vi "난수플롯이벤트.vi"() -> ()   [LabVIEW 2014]
panel:
  in  "정지":bool
  out "웨이브폼 차트":dbl(graph)
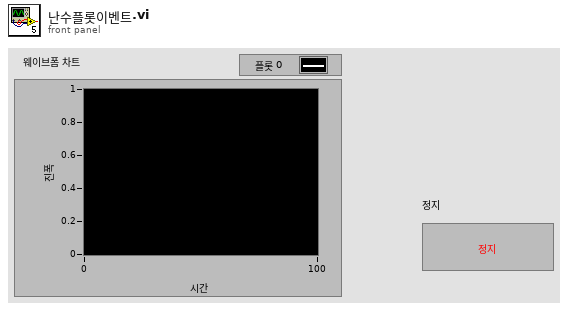
[diagram p1: front panel]
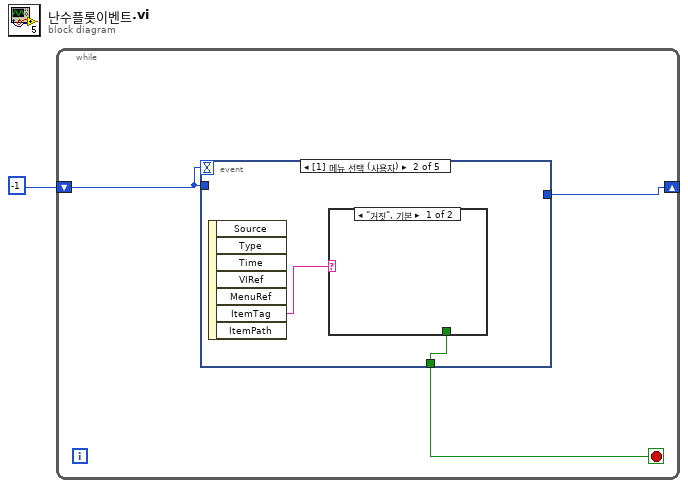
[diagram p0: block diagram]
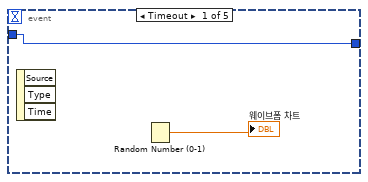
[diagram p2: hidden frame]
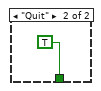
[diagram p3: hidden frame]
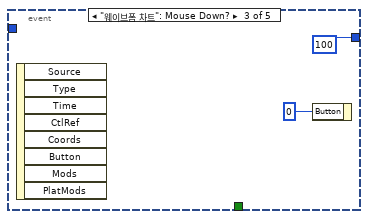
[diagram p4: hidden frame]
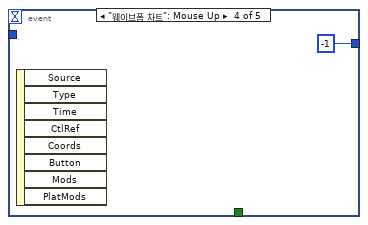
[diagram p5: hidden frame]
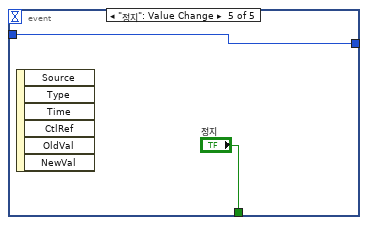
[diagram p6: hidden frame]
diagram:
  n1 = while {
    shift-right: [w3] -> _
    shift-left: -1 -> [w2]
    stop <- w4 stop-if-true
    n2 = event shown="[1] 메뉴 선택 (사용자)" {
      selector: _ -> [_ _ _ _ _]
      dyn-events: _ -> [_ _ _ _ _]
      timeout: w2 -> [_ _ _ _ _]
      tunnel: [_ w7 _ _ "정지"] -> w4
      tunnel: [w5 _ 100 -1 w13] -> w3
      tunnel: w2 -> [w5 _ _ _ w13]
      event Timeout {
        n3 = event-data() -> ()  [unwired: 1 in, 3 out]
        n4 = Random Number (0-1)() -> (number: 0 to 1=→"웨이브폼 차트":dbl)
      }
      event Menu Selection (User) {
        n5 = event-data() -> ("ItemTag"=w8:string)  [unwired: 1 in, 6 out]
        n6 = case shown="\"거짓\", 기본" w8 {
          tunnel: [_ TRUE] -> w7
          frame "거짓", Default {
          }
          frame "Quit" {
          }
        }
      }
      event "웨이브폼 차트": Mouse Down? {
        n7 = event-data() -> ()  [unwired: 1 in, 8 out]
        n8 = event-data("Button"=u16 0 ("버튼")) -> ()  [unwired: 1 in, 1 out]
      }
      event "웨이브폼 차트": Mouse Up {
        n9 = event-data() -> ()  [unwired: 1 in, 8 out]
      }
      event "정지": Value Change {
        n10 = event-data() -> ()  [unwired: 1 in, 6 out]
      }
    }
  }
